vi "H5Ovisit_by_name.vi"(0 "Location Ref":T1, 1 "Index Type":T3 items=["H5_INDEX_UNKNOWN"=-1, "H5_INDEX_NAME"=0, "H5_INDEX_CRT_ORDER"=1], 2 "Order":T2 items=["H5_ITER_UNKNOWN"=-1, "H5_ITER_INC"=0, "H5_ITER_DEC"=1], 5 "Object Name":string=".", 7 "User data":variant, 11 "error in (no error)":errorcluster, 12 "Callback VI Ref":refnum<vi>, 13 "lapl_id":T1) -> (4 "Location Ref out":T1, 8 "User data out":variant, 15 "error out":errorcluster)   [LabVIEW 2017]
doc: "Recursively visits all objects starting from a specified object."
uses:
  <vilib>/UPVI/lvhdf5/library.llb/HDF5 Ref.ctl
  <vilib>/UPVI/lvhdf5/object.llb/H5O_info_t.ctl
  <vilib>/UPVI/lvhdf5/object.llb/H5O_type_t.ctl
  <vilib>/UPVI/lvhdf5/object.llb/H5O_hdr_info_t.ctl
  <vilib>/UPVI/lvhdf5/library.llb/H5_ih_info_t.ctl
  <vilib>/UPVI/lvhdf5/library.llb/H5_index_t.ctl
  <vilib>/UPVI/lvhdf5/library.llb/H5_iter_order_t.ctl
  <vilib>/UPVI/lvhdf5/h5helper.dll
panel:
  in  "Event Data Type":T8 {"info"."H5O_hdr_info_t"."mesg"."shared" format="%.0x"; "info"."H5O_hdr_info_t"."mesg"."present" format="%.0x"; "info"."H5O_hdr_info_t"."flags" format="%.0x"; "info"."type" items=["H5O_TYPE_UNKNOWN"=-1, "H5O_TYPE_GROUP"=0, "H5O_TYPE_DATASET"=1, "H5O_TYPE_NAMED_DATATYPE"=2]}
  # "LVHDF5 Toolkit\nCopyright (c) 2005-2013 by Jason D. Sommerville\nCopyright (c) 2014-2015 by UPVI, LLC.\n\nThis use and distribution of this file is governed by the terms found in \nLICENSE.txt distributed with this toolkit and installed at\n <user.lib>\\_lvhdf5\\LICENSE.txt"
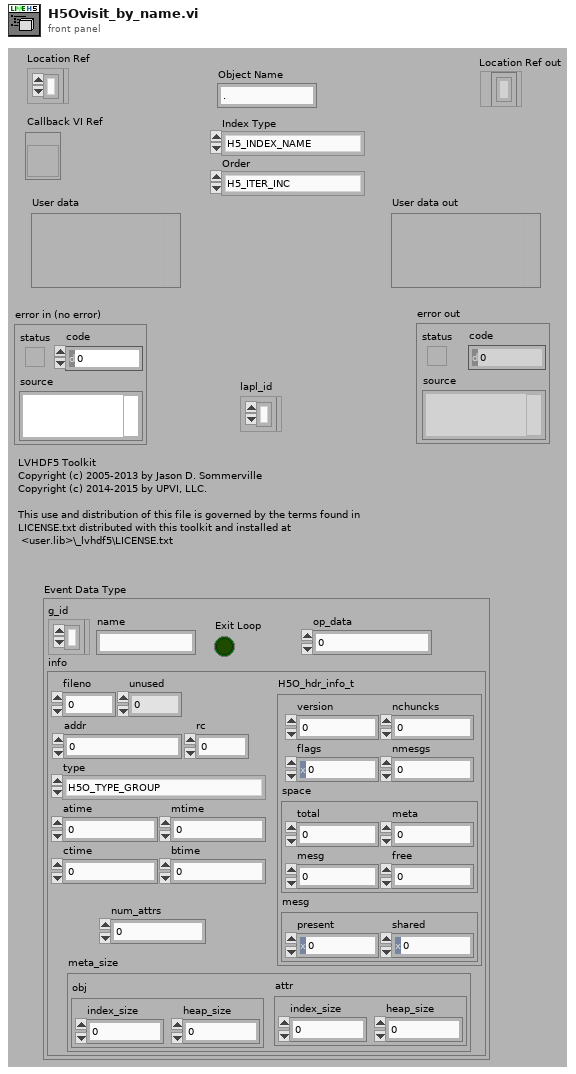
[diagram p1: front panel]
types:
  T1 = typedef "HDF5 Ref.ctl" = refnum<k1>
  T2 = typedef "H5_iter_order_t.ctl" = i32
  T3 = typedef "H5_index_t.ctl" = i32
  T4 = typedef "H5O_info_t.ctl" = cluster{"fileno":u32, "unused":u32, "addr":u64, "type":T5, "rc":u32, "atime":i64, "mtime":i64, "ctime":i64, "btime":i64, "num_attrs":i64, "H5O_hdr_info_t":T6, "meta_size":cluster{"obj":T7, "attr":T7}}
  T5 = typedef "H5O_type_t.ctl" = i32
  T6 = typedef "H5O_hdr_info_t.ctl" = cluster{"version":u32, "nmesgs":u32, "nchuncks":u32, "flags":u32, "space":cluster{"total":u64, "meta":u64, "mesg":u64, "free":u64}, "mesg":cluster{"present":u64, "shared":u64}}
  T7 = typedef "H5_ih_info_t.ctl" = cluster{"index_size":u64, "heap_size":u64}
  T8 = cluster{"g_id":T1, "name":string, "info":T4, "Exit Loop":bool, "op_data":u64}
  T9 = typedef "LVH5O_info_t.ctl" = cluster{"fileno":u32, "addr":u64, "type":T5, "rc":u32, "atime":timestamp, "mtime":timestamp, "ctime":timestamp, "btime":timestamp, "num_attrs":i64, "H5O_hdr_info_t":T6, "meta_size":cluster{"obj":T7, "attr":T7}}
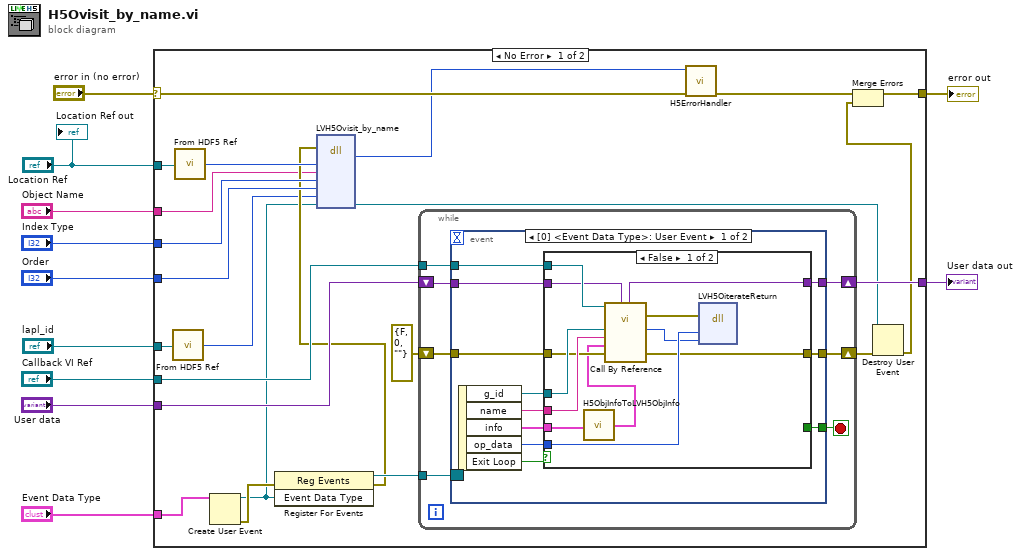
[diagram p0: block diagram]
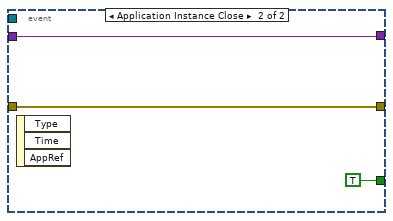
[diagram p3: hidden frame]
diagram:
  n1 = case shown="No Error" "error in (no error)" {
    selector: "error in (no error)" -> [w34 w72]
    tunnel: [w23 w72] -> w10
    tunnel: "Location Ref" -> [w32 _]
    tunnel: "Callback VI Ref" -> [w30 _]
    tunnel: "User data" -> [w29 w71]
    tunnel: "Event Data Type" -> [w26 _]
    tunnel: [w27 w71] -> w6
    tunnel: "Index Type" -> [w19 _]
    tunnel: "Order" -> [w18 _]
    tunnel: "Object Name" -> [w16 _]
    tunnel: "lapl_id" -> [w15 _]
    frame No Error {
      n2 = call <vilib>:"From HDF5 Ref.vi"("HDF5 Ref"=w15) -> ("I32"=w14:i32)
      n3 = call <vilib>:"From HDF5 Ref.vi"("HDF5 Ref"=w32) -> ("I32"=w25:i32)
      n4 = Create User Event(user event datatype=w26) -> (user event=w12:refnum<user-event>, error out=w31:errorcluster)  [unwired: 1 in]
      n5 = register-events(error in=w31, w12) -> (reference out=w28:refnum<event-registration>, error out=w17:errorcluster)  [unwired: 1 in]
      n6 = dll-call lib="C:/Program Files/National Instruments/LabVIEW 2017/vi.lib/UPVI/lvhdf5/h5helper.dll" fn="LVH5Ovisit_by_name" label="LVH5Oiterate_by_name"(error in=w17, "grp_id"=w25, "grp_name"=w16, "index_type"=w19, "order"=w18, "lapl_id"=w14, "lvevt"=w12) -> ("return type"=w33:i32, "lvevt"=w20:refnum<user-event>)  [unwired: 7 in, 2 out]
      n7 = while {
        tunnel: w28 -> [w41]
        tunnel: w30 -> [w40]
        shift-right: [w38] -> w27
        shift-left: w29 -> [w39]
        shift-right: [w36] -> w22
        shift-left: errorcluster {"status"=FALSE, "code"=0, "source"=""} ("error out") -> [w35]
        stop <- w37 stop-if-true
        n8 = event shown="[0] <Event Data Type>: User Event" {
          selector: w41 -> [_ _]
          dyn-events: _ -> [_ _]
          timeout: _ -> [_ _]
          tunnel: w40 -> [w52 _]
          tunnel: w39 -> [w48 w69]
          tunnel: [w47 w69] -> w38
          tunnel: [w46 TRUE] -> w37
          tunnel: [w43 w68] -> w36
          tunnel: w35 -> [w42 w68]
          event User Event {
            n9 = event-data() -> ("g_id"=w51:T1, "name"=w50:string, "info"=w49:T4, "op_data"=w44:u64, "Exit Loop"=w45:bool)  [unwired: 1 in]
            n10 = case shown="False" w45 {
              selector: w45 -> [_ w66]
              tunnel: w52 -> [w64 _]
              tunnel: w51 -> [w63 _]
              tunnel: w50 -> [w62 _]
              tunnel: w49 -> [w54 _]
              tunnel: w48 -> [w61 w67]
              tunnel: [w60 w67] -> w47
              tunnel: [_ w66] -> w46
              tunnel: w44 -> [w58 _]
              tunnel: [w56 w65] -> w43
              tunnel: w42 -> [w55 w65]
              frame False {
                n11 = call <vilib>:"H5ObjInfoToLVH5ObjInfo.vi"("H5O_info_t"=w54) -> ("LVH5O_info_t"=w53:T9)
                n12 = call-by-ref "?"(reference=w64, "op_data"=w61, "error in (no error)"=w55, "info"=w53, "name"=w62, "g_id"=w63) -> (error out=w59:errorcluster, 0:"error out"=w56:errorcluster, "Stop"=w57:i32, "op_data out"=w60:variant)  [unwired: 5 in, 1 out]
                n13 = dll-call lib="C:/Program Files/National Instruments/LabVIEW 2017/vi.lib/UPVI/lvhdf5/h5helper.dll" fn="LVH5OiterateReturn"(error in=w59, "op_data"=w58, "result"=w57) -> ()  [unwired: 5 in, 2 out]
              }
              frame True {
              }
            }
          }
          event Application Instance Close {
            n14 = event-data() -> ()  [unwired: 1 in, 3 out]
          }
        }
      }
      n15 = call <vilib>:"H5ErrorHandler.vi"("error in (no error)"=w34, "herr_t"=w33) -> ("error out"=w24:errorcluster)  [unwired: 3 in, 4 out]
      n16 = Destroy User Event(user event=w20, error in=w22) -> (error out=w21:errorcluster)
      n17 = Merge Errors(w24, w21) -> (w23:errorcluster)
    }
    frame Error {
    }
  }
  "error out" <- w10
  "User data out" <- w6
  "Location Ref out" <- "Location Ref"
